vi "MSG.vi"(0 "System no.":i32=1 min=1 max=4 step=1, 3 "Message":string, 5 "error in":errorcluster) -> (19 "error out":errorcluster)   [LabVIEW 2026]
doc: "Displays a message on the controller display."
panel:
  # "Displays a message on the controller display."
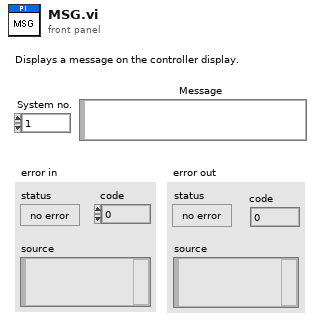
[diagram p1: front panel]
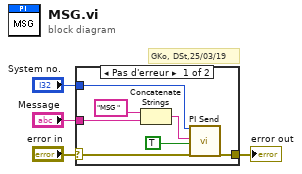
[diagram p0: block diagram]
diagram:
  # "GKo, DSt,25/03/19"
  n1 = case shown="Pas d'erreur" "error in" {
    selector: "error in" -> [w5 w12]
    tunnel: "System no." -> [w9 _]
    tunnel: "Message" -> [w7 _]
    tunnel: [w6 w12] -> w2
    frame No Error {
      n2 = Concatenate Strings("MSG ", w7) -> (w8:string)
      n3 = call "PI Send.vi"("System no."=w9, "String to send"=w8, "Attach termination char.?"=TRUE ("Attach Linefeed?"), "error in"=w5) -> ("error out"=w6:errorcluster)  [unwired: 2 in, 13 out]
    }
    frame Error {
    }
  }
  "error out" <- w2
